vi "Bataille.vi"() -> ()   [LabVIEW 2019]
uses:
  C:/Users/benjamin.mestre/Downloads/BatailleLV/BatailleLibrairie/BatailleLibrairie/bin/Debug/BatailleLibrairie.dll
  BatailleLibrairie/BatailleLibrairie/bin/Debug/BatailleLibrairie.dll
panel:
  out "Nom Gagnant":string
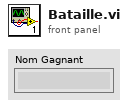
[diagram p1: front panel]
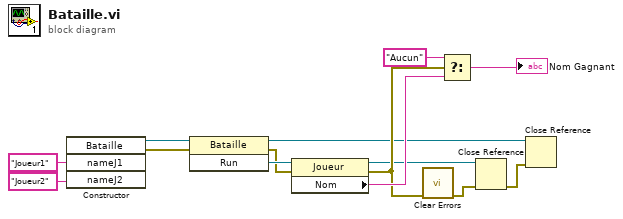
[diagram p0: block diagram]
diagram:
  n1 = constructor class="Bataille"("nameJ1"="Joueur1", "nameJ2"="Joueur2") -> (reference out=w1:refnum<k24>, error out=w8:errorcluster)  [unwired: 3 in, 3 out]
  n2 = invoke class="Bataille" method="Run"(reference=w1, error in=w8) -> (reference out=w2:refnum<k24>, error out=w7:errorcluster, "Run"=w12:refnum<k24>)  [unwired: 1 in]
  n3 = property class="Joueur"(reference=w12, error in=w7) -> (reference out=w4:refnum<k24>, error out=w6:errorcluster, "Nom"=w11:string)
  n4 = call <vilib>:"Clear Errors.vi"("error in (no error)"=w6) -> ("error out"=w5:errorcluster)  [unwired: 5 in, 1 out]
  n5 = Select(t="Aucun" ("cas vrai"), s=w6, f=w11) -> (s? t:f=→"Nom Gagnant":string)
  n6 = Close Reference(reference=w4, error in (no error)=w5) -> (error out=w3:errorcluster)
  n7 = Close Reference(reference=w2, error in (no error)=w3) -> ()  [unwired: 1 out]
